vi "Create_AO_POLAR_WF.vi"(8 "error in":errorcluster) -> (0 "error out":errorcluster)   [LabVIEW 2025]
uses:
  <vilib>/Waveform/WDTOps.llb/WDT Append Waveforms DBL.vi
panel:
  out "Illumination analog waveforms":waveform(dbl)(graph) caption="Output Waveform"
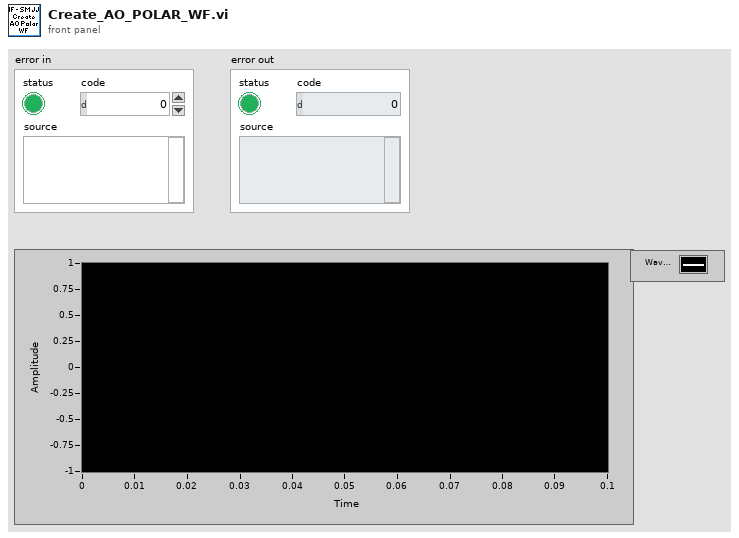
[diagram p1: front panel]
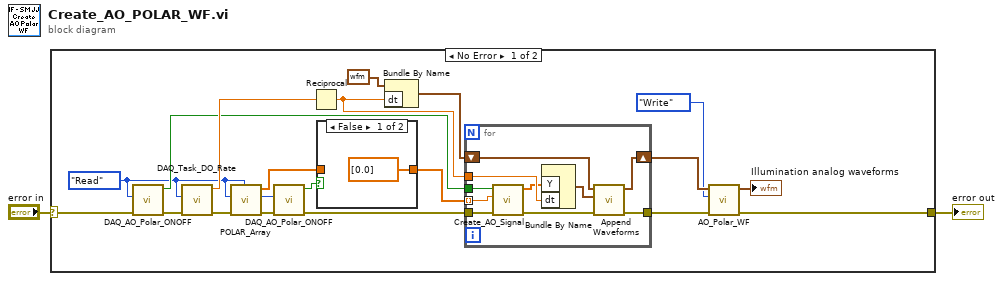
[diagram p0: block diagram]
diagram:
  n1 = case shown="No Error" "error in" {
    selector: "error in" -> [w21 w34]
    tunnel: [w20 w34] -> w1
    frame No Error {
      w3 = enum16{"Init", "Write", "Read"}."Read" ("Action")
      n2 = call "DAQ_AO_Polar_ONOFF.vi"("error in"=w21, "Action"=w3) -> ("error out"=w19:errorcluster, "ON / OFF"=w10:bool)  [unwired: 8 in]
      n3 = call "DAQ_Task_DO_Rate.vi"("error in"=w19, "Action"=w3) -> ("error out"=w17:errorcluster, "DO_Rate"=w18:dbl)  [unwired: 8 in]
      n4 = call "POLAR_Array.vi"("error in"=w17, "Action"=w3) -> ("error out"=w8:errorcluster, "Pockels_Array"=w5:dbl[])  [unwired: 8 in]
      n5 = call "DAQ_AO_Polar_ONOFF.vi"("error in"=w8, "Action"=w3) -> ("error out"=w7:errorcluster, "ON / OFF"=w6:bool)  [unwired: 8 in]
      n6 = Reciprocal(x=w18) -> (1/x=w14:dbl)
      n7 = case shown="False" w6 {
        tunnel: w5 -> [_ w23]
        tunnel: [dbl[] [0.0] ("Pockels_Array") w23] -> w4
        frame False {
        }
        frame True {
        }
      }
      n8 = Bundle By Name(cluster=waveform(dbl) {"t0"=timestamp(0 s since 1904-01-01), "dt"=0.001, "Y"=[]} ("waveform out"), "dt"=w14) -> (w13:waveform(dbl))
      n9 = for {
        tunnel: [w25] -> w11
        tunnel: w10 -> [w33]
        tunnel: w14 -> [w32]
        tunnel: w4 -> [w30] mode=indexing
        tunnel: w7 -> [w29]
        shift-right: [w26] -> w12
        shift-left: w13 -> [w27]
        n10 = call "Create_AO_Signal.vi"("error in"=w29, "AO Amplitude"=w30, "ON / OFF"=w33) -> ("error out"=w28:errorcluster, "WF"=w31:dbl[])  [unwired: 7 in]
        n11 = Bundle By Name("Y"=w31, "dt"=w32) -> (w24:waveform(dbl))  [unwired: 1 in]
        n12 = call-poly <vilib>:"Append Waveforms.vi"("error in (no error)"=w28, "waveform B"=w24, "waveform A"=w27) -> ("error out"=w25:errorcluster, "waveform out"=w26:waveform(dbl))  [unwired: 7 in]
      }
      n13 = call "AO_Polar_WF.vi"("error in"=w11, "Action"=enum16{"Init", "Write", "Read"}."Write", "AO Polar WF"=w12) -> ("error out"=w20:errorcluster, "AO Poalr WF"=→"Illumination analog waveforms":waveform(dbl))  [unwired: 7 in]
    }
    frame Error {
    }
  }
  "error out" <- w1
